vi "Config - access language vision ini file.vi"(5 ".ini Controller":enum16{"Read", "Write"}(ring), 6 "Language":T1, 8 "error in":errorcluster, 10 "English":T2={"Home"="Home", "Test Setup"="Setup", "Run Test"="Test", "Configure"="Config", "Hardware Viewer"="Viewer", "Review Test"="Review", "Report"="Folder Path:", "Exit"="Exit", "Device Connected?"="Device Connected?", "Test in Progress?"="Test in Progress?", "Simulate?"="Simulate?", "Device Type 1"="Corrugation Analysis Trolley", "Device Type 2"="Bi-Corrugation Analysis Trolley", "Device Type 3"="Bi-Corrugation Analysis Trolley", "Device Type 4"="Bi-Corrugation Analysis Trolley", "Device Type 5"="Bi-Corrugation Analysis Trolley", "Device Type 6"="Bi-Corrugation Analysis Trolley", "Device Type 7"="Bi-Corrugation Analysis Trolley", "Software Version"="Version", "Support"="Software by RailMeasurement Limited - Cambridge - UK - support@railmeasurement.com", "Operator"="Operator:", "Test Description"="Description:", "Line"="Description:", "Test Folder Path"="Folder Path:", "Test Folder Path RCA"="Folder Path:", "Start Position"="Start Position:", "Sensor Position"="Sensor Position:", "Sensor A Position"="Sensor A Position:", "Sensor B Position"="Sensor B Position:", "Visible Chart Distance"="Sensor B Position:", "Rail Side"="Rail Side:", "Rail A Side"="Rail A Side:", "Distance Direction"="Distance Direction:", "Start"="Start:", "Distance Travelled"="Distance Travelled:", "Current Position"="Current Position:", "Stop Test"="Stop", "Pause Test"="Save", "Displacement"="Displacement", "Position"="Position", "Sensor Calibration"="Sensor Calibration:", "Sensor A Calibration"="Sensor A Calibration:", "Sensor B Calibration"="Sensor B Calibration:", "Encoder Spacing"="Encoder Spacing:", "Sampling Distance"="Sampling Distance:", "Tacho Pulses/Rev"="Sensor Calibration:", "Wheel Diameter"="Sensor A Calibration:", "Sampling Distances"=["1mm", "2mm"], "Distance Unit"="Distance in:", "Distance Units"=["Kilometres", "miles & chains", "metres", "stations", "miles"], "Swap Direction"="Swap Direction at Run End?", "Language"="Language", "Device Resolution"="Save", "Device Resolutions"=["Kilometres", "miles & chains", "metres", "stations", "miles"], "Detect Change in Direction"="Save", "Save Config"="Save", "Encoder Data"="Encoder Data", "Sensor Data"="Sensor Data", "Sensor A Data"="Sensor A Data", "Sensor B Data"="Sensor B Data", "Voltage"="Voltage", "Time (m:s)"="Time (m:s)", "Unit mm/s/V"="(mm/s)/V", "Unit mm"="mm", "Unit km"="km", "Unit m"="m", "Start Test Message"="m", "Stop Test Message"="km", "Exit Message"="mm", "File Exists Message"="mm", "File Path Invalid Message"="mm", "Combine Error"="mm", "Combine Success"="mm", "Roller Comp Error"="mm", "Test Folder Path (Live)"="mm", "Folder Error"="Sensor B Position:", "Enc Count"="Setup", "Run Start"="mm", "Run End"="mm", "Date"="mm", "Train"="Sensor B Position:", "Location"="Setup", "Notes"="mm", "Heading_1"="mm", "Heading_2"="mm", "Left Rail"="Sensor B Position:", "Right Rail"="Setup", "Left Exclusions"="mm", "Right Exclusions"="mm", "Settings"="mm", "Wavelength Ranges"="Sensor B Position:", "Y-Axis Limits"="Setup", "Exc Limits"="Sensor B Position:", "Other Settings"="Setup", "Distance/Page"="mm", "Distance/Pages"=["Kilometres", "miles & chains", "metres", "stations", "miles"], "Gridlines"="mm", "Report Tolerance"="mm", "Manual Cut"="Sensor B Position:", "Plot Colour"="Distance in:", "Plot Colours"=["Kilometres", "miles & chains", "metres", "stations", "miles"], "EN Standard"="mm", "RiL Standard"="mm", "Custom Standard"="mm", "Resolution"="Distance in:", "Resolutions"=["Kilometres", "miles & chains", "metres", "stations", "miles"], "Exceedence Header"="mm", "Distance (km)"="mm", "Left (%)"="mm", "Right (%)"="Distance in:", "Page"="Distance in:", "Align"="mm", "Main"="mm", "Comparison"="Distance in:", "Offset"="Distance in:", "From"="Distance in:", "To"="Distance in:", "Of"="Distance in:", "File"="mm", "Load New"="mm", "Load Comparison"="Distance in:", "Discard Comparison"="Distance in:", "Print Current Page"="Distance in:", "Print All Pages"="Distance in:", "Print Exceedence Report"="Distance in:", "Plot Main"="Distance in:", "No Comparison Data to Align"="Distance in:", "Run Load Error"="Distance in:", "Report Load Error"="Distance in:", "Cut"="Distance in:", "Remove"="Distance in:", "Config Settings Unsaved"="Distance in:", "Acquisition Paused"="Distance in:", "Please Select One Option Below"="Distance in:", "RCA is Now Stationary"="Distance in:", "Reporting Setting"="Distance in:", "Main Abbreviated"="Distance in:", "Comparison Abbreviated"="Distance in:", "Exceedence Abbreviated"="Distance in:", "Align Comparison"="Distance in:", "Rail Corrugation Analyser Reporting"="Distance in:", "Show Exc. % in Graph"="Distance in:", "Evaluate Sections <100m"="Distance in:", "Evaluate Sections <0.062mile"="Distance in:", "Section Too Short for Evaluation"="Distance in:", "Language Change Prompt"="Distance in:", "Show All"="Distance in:", "Sections_km"="Distance in:", "Sections_mi"="Distance in:", "Vision"="Distance in:", "Vision Report"="Distance in:", "Vision Display"="Distance in:", "Vision Displays"=["Kilometres", "miles & chains", "metres", "stations", "miles"], "Save Images"="Distance in:", "Image Frequency"="Distance in:", "Section"="Distance in:", "Brightness"="Distance in:", "Contrast"="Distance in:", "Shadow"="Distance in:", "Sharpened"="Distance in:", "Apply to all Images"="Distance in:", "Reset"="Distance in:", "Are you sure"="Distance in:", "Image Processing"="Distance in:", "Save Video"="Distance in:", "Image Offset"="Distance in:", "Camera Mode"="Distance in:", "Camera Modes"=["Kilometres", "miles & chains", "metres", "stations", "miles"], "Copy Page"="Distance in:", "Copy Graphs"="Distance in:", "Camera Mode Change Prompt"="Distance in:", "Camera_1 Missing"="Distance in:", "Camera_2 Missing"="Distance in:", "Cameras Missing"="Distance in:", "Camera Setup"="Distance in:", "Camera_1 Connection Error"="Distance in:", "Camera_2 Connection Error"="Distance in:", "Cameras Connection Error"="Distance in:", "No GPS"="Distance in:", "No Signal"="Distance in:", "Camera_1 Connected"="Distance in:", "Camera_1 Not Connected"="Distance in:", "Camera_2 Connected"="Distance in:", "Camera_2 Not Connected"="Distance in:", "Start Position at 0m?"="Distance in:", "Continue"="Distance in:", "New Test, Same Direction"="Distance in:", "New Test, Opposite Direction"="Distance in:", "Stop and Save"="Distance in:", "Live Corrug Estimate"="Distance in:", "Wavelength Corrug"="Distance in:", "Distance Corrug "="Distance in:", "Update Corrug"="Distance in:", "Company"="Distance in:", "Ref Profile "="Distance in:", "Company_Report"="Distance in:", "Ref Profile_Report"="Distance in:", "Heading_1_RVHR"="Distance in:", "Heading_2_RVHR"="Distance in:", "Remove Feature"="Distance in:", "Feature Type"="Sampling Distance:", "Feature Types"=["1mm", "2mm"], "AI Not Ready"="Sampling Distance:"}, 11 "Config File Ref":T3=refnum) -> (0 "error out":errorcluster, 2 "HLC Controls Out":T2={"Home"="Home", "Test Setup"="Setup", "Run Test"="Test", "Configure"="Config", "Hardware Viewer"="Viewer", "Review Test"="Review", "Report"="Folder Path:", "Exit"="Exit", "Device Connected?"="Device Connected?", "Test in Progress?"="Test in Progress?", "Simulate?"="Simulate?", "Device Type 1"="Corrugation Analysis Trolley", "Device Type 2"="Bi-Corrugation Analysis Trolley", "Device Type 3"="Bi-Corrugation Analysis Trolley", "Device Type 4"="Bi-Corrugation Analysis Trolley", "Device Type 5"="Bi-Corrugation Analysis Trolley", "Device Type 6"="Bi-Corrugation Analysis Trolley", "Device Type 7"="Bi-Corrugation Analysis Trolley", "Software Version"="Version", "Support"="Software by RailMeasurement Limited - Cambridge - UK - support@railmeasurement.com", "Operator"="Operator:", "Test Description"="Description:", "Line"="Description:", "Test Folder Path"="Folder Path:", "Test Folder Path RCA"="Folder Path:", "Start Position"="Start Position:", "Sensor Position"="Sensor Position:", "Sensor A Position"="Sensor A Position:", "Sensor B Position"="Sensor B Position:", "Visible Chart Distance"="Sensor B Position:", "Rail Side"="Rail Side:", "Rail A Side"="Rail A Side:", "Distance Direction"="Distance Direction:", "Start"="Start:", "Distance Travelled"="Distance Travelled:", "Current Position"="Current Position:", "Stop Test"="Stop", "Pause Test"="Save", "Displacement"="Displacement", "Position"="Position", "Sensor Calibration"="Sensor Calibration:", "Sensor A Calibration"="Sensor A Calibration:", "Sensor B Calibration"="Sensor B Calibration:", "Encoder Spacing"="Encoder Spacing:", "Sampling Distance"="Sampling Distance:", "Tacho Pulses/Rev"="Sensor Calibration:", "Wheel Diameter"="Sensor A Calibration:", "Sampling Distances"=["1mm", "2mm"], "Distance Unit"="Distance in:", "Distance Units"=["Kilometres", "miles & chains", "metres", "stations", "miles"], "Swap Direction"="Swap Direction at Run End?", "Language"="Language", "Device Resolution"="Save", "Device Resolutions"=["Kilometres", "miles & chains", "metres", "stations", "miles"], "Detect Change in Direction"="Save", "Save Config"="Save", "Encoder Data"="Encoder Data", "Sensor Data"="Sensor Data", "Sensor A Data"="Sensor A Data", "Sensor B Data"="Sensor B Data", "Voltage"="Voltage", "Time (m:s)"="Time (m:s)", "Unit mm/s/V"="(mm/s)/V", "Unit mm"="mm", "Unit km"="km", "Unit m"="m", "Start Test Message"="m", "Stop Test Message"="km", "Exit Message"="mm", "File Exists Message"="mm", "File Path Invalid Message"="mm", "Combine Error"="mm", "Combine Success"="mm", "Roller Comp Error"="mm", "Test Folder Path (Live)"="mm", "Folder Error"="Sensor B Position:", "Enc Count"="Setup", "Run Start"="mm", "Run End"="mm", "Date"="mm", "Train"="Sensor B Position:", "Location"="Setup", "Notes"="mm", "Heading_1"="mm", "Heading_2"="mm", "Left Rail"="Sensor B Position:", "Right Rail"="Setup", "Left Exclusions"="mm", "Right Exclusions"="mm", "Settings"="mm", "Wavelength Ranges"="Sensor B Position:", "Y-Axis Limits"="Setup", "Exc Limits"="Sensor B Position:", "Other Settings"="Setup", "Distance/Page"="mm", "Distance/Pages"=["Kilometres", "miles & chains", "metres", "stations", "miles"], "Gridlines"="mm", "Report Tolerance"="mm", "Manual Cut"="Sensor B Position:", "Plot Colour"="Distance in:", "Plot Colours"=["Kilometres", "miles & chains", "metres", "stations", "miles"], "EN Standard"="mm", "RiL Standard"="mm", "Custom Standard"="mm", "Resolution"="Distance in:", "Resolutions"=["Kilometres", "miles & chains", "metres", "stations", "miles"], "Exceedence Header"="mm", "Distance (km)"="mm", "Left (%)"="mm", "Right (%)"="Distance in:", "Page"="Distance in:", "Align"="mm", "Main"="mm", "Comparison"="Distance in:", "Offset"="Distance in:", "From"="Distance in:", "To"="Distance in:", "Of"="Distance in:", "File"="mm", "Load New"="mm", "Load Comparison"="Distance in:", "Discard Comparison"="Distance in:", "Print Current Page"="Distance in:", "Print All Pages"="Distance in:", "Print Exceedence Report"="Distance in:", "Plot Main"="Distance in:", "No Comparison Data to Align"="Distance in:", "Run Load Error"="Distance in:", "Report Load Error"="Distance in:", "Cut"="Distance in:", "Remove"="Distance in:", "Config Settings Unsaved"="Distance in:", "Acquisition Paused"="Distance in:", "Please Select One Option Below"="Distance in:", "RCA is Now Stationary"="Distance in:", "Reporting Setting"="Distance in:", "Main Abbreviated"="Distance in:", "Comparison Abbreviated"="Distance in:", "Exceedence Abbreviated"="Distance in:", "Align Comparison"="Distance in:", "Rail Corrugation Analyser Reporting"="Distance in:", "Show Exc. % in Graph"="Distance in:", "Evaluate Sections <100m"="Distance in:", "Evaluate Sections <0.062mile"="Distance in:", "Section Too Short for Evaluation"="Distance in:", "Language Change Prompt"="Distance in:", "Show All"="Distance in:", "Sections_km"="Distance in:", "Sections_mi"="Distance in:", "Vision"="Distance in:", "Vision Report"="Distance in:", "Vision Display"="Distance in:", "Vision Displays"=["Kilometres", "miles & chains", "metres", "stations", "miles"], "Save Images"="Distance in:", "Image Frequency"="Distance in:", "Section"="Distance in:", "Brightness"="Distance in:", "Contrast"="Distance in:", "Shadow"="Distance in:", "Sharpened"="Distance in:", "Apply to all Images"="Distance in:", "Reset"="Distance in:", "Are you sure"="Distance in:", "Image Processing"="Distance in:", "Save Video"="Distance in:", "Image Offset"="Distance in:", "Camera Mode"="Distance in:", "Camera Modes"=["Kilometres", "miles & chains", "metres", "stations", "miles"], "Copy Page"="Distance in:", "Copy Graphs"="Distance in:", "Camera Mode Change Prompt"="Distance in:", "Camera_1 Missing"="Distance in:", "Camera_2 Missing"="Distance in:", "Cameras Missing"="Distance in:", "Camera Setup"="Distance in:", "Camera_1 Connection Error"="Distance in:", "Camera_2 Connection Error"="Distance in:", "Cameras Connection Error"="Distance in:", "No GPS"="Distance in:", "No Signal"="Distance in:", "Camera_1 Connected"="Distance in:", "Camera_1 Not Connected"="Distance in:", "Camera_2 Connected"="Distance in:", "Camera_2 Not Connected"="Distance in:", "Start Position at 0m?"="Distance in:", "Continue"="Distance in:", "New Test, Same Direction"="Distance in:", "New Test, Opposite Direction"="Distance in:", "Stop and Save"="Distance in:", "Live Corrug Estimate"="Distance in:", "Wavelength Corrug"="Distance in:", "Distance Corrug "="Distance in:", "Update Corrug"="Distance in:", "Company"="Distance in:", "Ref Profile "="Distance in:", "Company_Report"="Distance in:", "Ref Profile_Report"="Distance in:", "Heading_1_RVHR"="Distance in:", "Heading_2_RVHR"="Distance in:", "Remove Feature"="Distance in:", "Feature Type"="Sampling Distance:", "Feature Types"=["1mm", "2mm"], "AI Not Ready"="Sampling Distance:"}, 3 "refnum out":T3)   [LabVIEW 2023]
doc: "This subVI reads initial config data from a .ini file to define the default UI.\n\nAuthor: D Keeling\nDate: 20/05/2012\nVersion: 1.0"
uses:
  <vilib>/Utility/config.llb/NI_LVConfig.lvlib
  <vilib>/Utility/config.llb/Config Data RefNum.ctl
  Controls/Language.ctl
  Controls/Language Vision Text Cluster.ctl
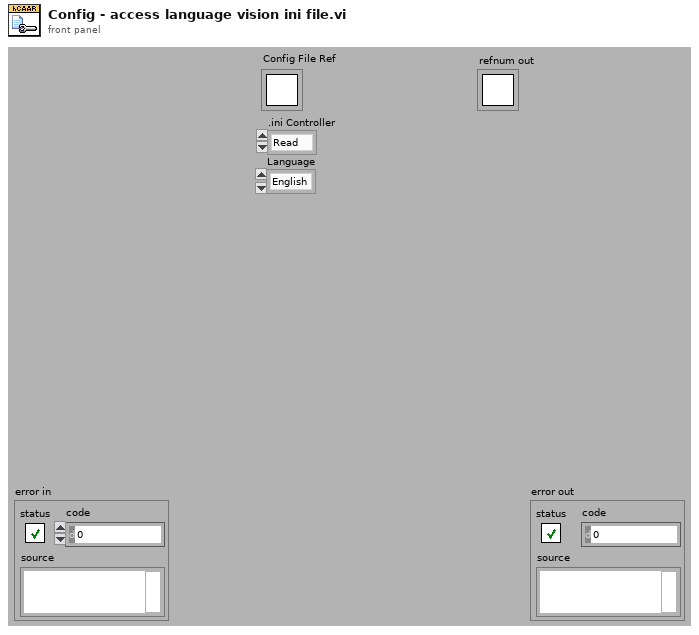
[diagram p1: front panel]
types:
  T1 = typedef "Language.ctl" = enum16{"English", "Chinese", "German"}
  T2 = typedef "Language Vision Text Cluster.ctl" = cluster{"Home":string, "Test Setup":string, "Run Test":string, "Configure":string, "Hardware Viewer":string, "Review Test":string, "Report":string, "Exit":string, "Device Connected?":string, "Test in Progress?":string, "Simulate?":string, "Device Type 1":string, "Device Type 2":string, "Device Type 3":string, "Device Type 4":string, "Device Type 5":string, "Device Type 6":string, "Device Type 7":string, "Software Version":string, "Support":string, "Operator":string, "Test Description":string, "Line":string, "Test Folder Path":string, "Test Folder Path RCA":string, "Start Position":string, "Sensor Position":string, "Sensor A Position":string, "Sensor B Position":string, "Visible Chart Distance":string, "Rail Side":string, "Rail A Side":string, "Distance Direction":string, "Start":string, "Distance Travelled":string, "Current Position":string, "Stop Test":string, "Pause Test":string, "Displacement":string, "Position":string, "Sensor Calibration":string, "Sensor A Calibration":string, "Sensor B Calibration":string, "Encoder Spacing":string, "Sampling Distance":string, "Tacho Pulses/Rev":string, "Wheel Diameter":string, "Sampling Distances":string[], "Distance Unit":string, "Distance Units":string[], "Swap Direction":string, "Language":string, "Device Resolution":string, "Device Resolutions":string[], "Detect Change in Direction":string, "Save Config":string, "Encoder Data":string, "Sensor Data":string, "Sensor A Data":string, "Sensor B Data":string, "Voltage":string, "Time (m:s)":string, "Unit mm/s/V":string, "Unit mm":string, "Unit km":string, "Unit m":string, "Start Test Message":string, "Stop Test Message":string, "Exit Message":string, "File Exists Message":string, "File Path Invalid Message":string, "Combine Error":string, "Combine Success":string, "Roller Comp Error":string, "Test Folder Path (Live)":string, "Folder Error":string, "Enc Count":string, "Run Start":string, "Run End":string, "Date":string, "Train":string, "Location":string, "Notes":string, "Heading_1":string, "Heading_2":string, "Left Rail":string, "Right Rail":string, "Left Exclusions":string, "Right Exclusions":string, "Settings":string, "Wavelength Ranges":string, "Y-Axis Limits":string, "Exc Limits":string, "Other Settings":string, "Distance/Page":string, "Distance/Pages":string[], "Gridlines":string, "Report Tolerance":string, "Manual Cut":string, "Plot Colour":string, "Plot Colours":string[], "EN Standard":string, "RiL Standard":string, "Custom Standard":string, "Resolution":string, "Resolutions":string[], "Exceedence Header":string, "Distance (km)":string, "Left (%)":string, "Right (%)":string, "Page":string, "Align":string, "Main":string, "Comparison":string, "Offset":string, "From":string, "To":string, "Of":string, "File":string, "Load New":string, "Load Comparison":string, "Discard Comparison":string, "Print Current Page":string, "Print All Pages":string, "Print Exceedence Report":string, "Plot Main":string, "No Comparison Data to Align":string, "Run Load Error":string, "Report Load Error":string, "Cut":string, "Remove":string, "Config Settings Unsaved":string, "Acquisition Paused":string, "Please Select One Option Below":string, "RCA is Now Stationary":string, "Reporting Setting":string, "Main Abbreviated":string, "Comparison Abbreviated":string, "Exceedence Abbreviated":string, "Align Comparison":string, "Rail Corrugation Analyser Reporting":string, "Show Exc. % in Graph":string, "Evaluate Sections <100m":string, "Evaluate Sections <0.062mile":string, "Section Too Short for Evaluation":string, "Language Change Prompt":string, "Show All":string, "Sections_km":string, "Sections_mi":string, "Vision":string, "Vision Report":string, "Vision Display":string, "Vision Displays":string[], "Save Images":string, "Image Frequency":string, "Section":string, "Brightness":string, "Contrast":string, "Shadow":string, "Sharpened":string, "Apply to all Images":string, "Reset":string, "Are you sure":string, "Image Processing":string, "Save Video":string, "Image Offset":string, "Camera Mode":string, "Camera Modes":string[], "Copy Page":string, "Copy Graphs":string, "Camera Mode Change Prompt":string, "Camera_1 Missing":string, "Camera_2 Missing":string, "Cameras Missing":string, "Camera Setup":string, "Camera_1 Connection Error":string, "Camera_2 Connection Error":string, "Cameras Connection Error":string, "No GPS":string, "No Signal":string, "Camera_1 Connected":string, "Camera_1 Not Connected":string, "Camera_2 Connected":string, "Camera_2 Not Connected":string, "Start Position at 0m?":string, "Continue":string, "New Test, Same Direction":string, "New Test, Opposite Direction":string, "Stop and Save":string, "Live Corrug Estimate":string, "Wavelength Corrug":string, "Distance Corrug ":string, "Update Corrug":string, "Company":string, "Ref Profile ":string, "Company_Report":string, "Ref Profile_Report":string, "Heading_1_RVHR":string, "Heading_2_RVHR":string, "Remove Feature":string, "Feature Type":string, "Feature Types":string[], "AI Not Ready":string}
  T3 = typedef "NI_LVConfig.lvlib/Config Data RefNum.ctl" = refnum<k1>
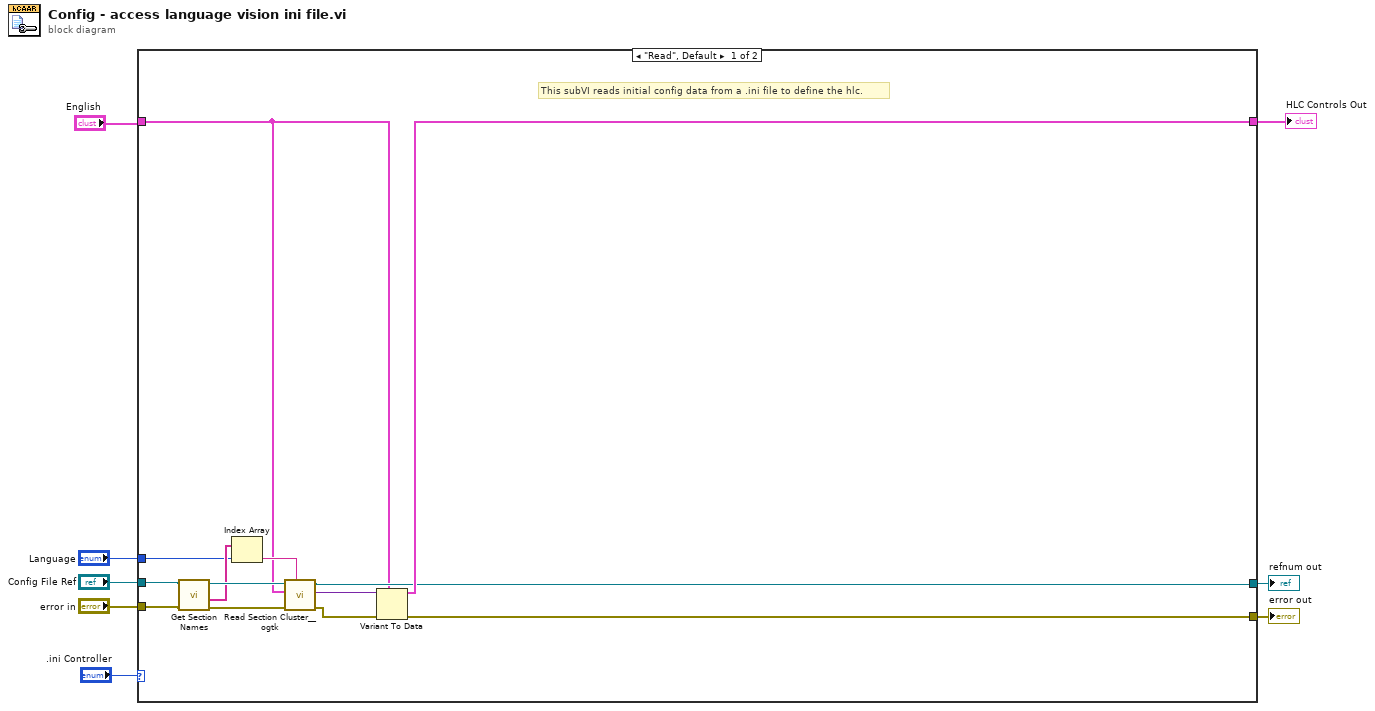
[diagram p0: block diagram]
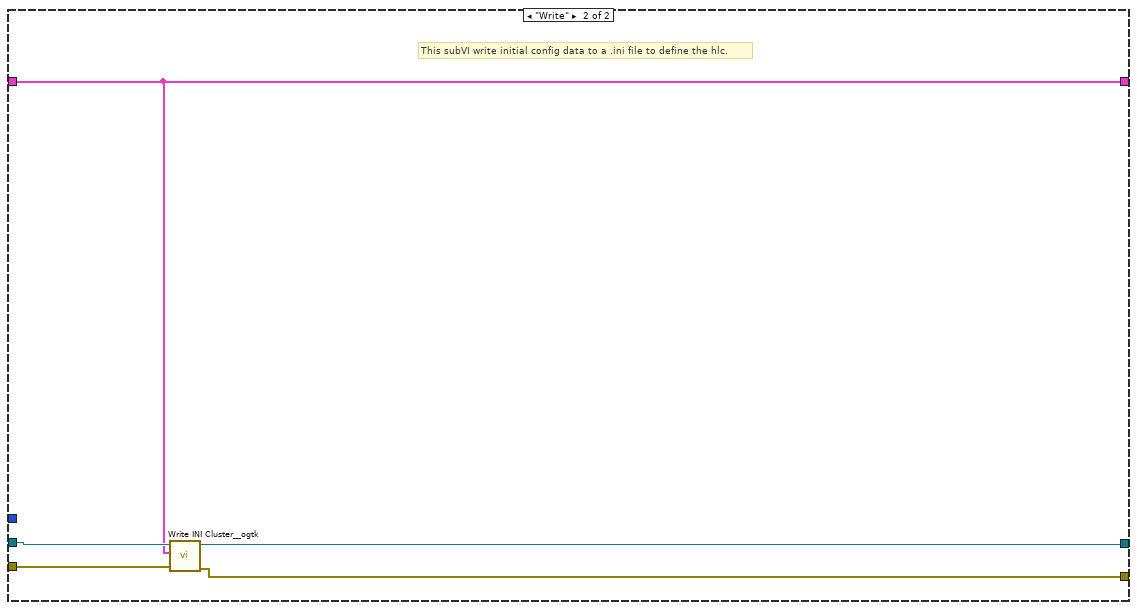
[diagram p2: hidden frame]
diagram:
  n1 = case shown="\"Read\", Default" ".ini Controller" {
    tunnel: [w21 w26] -> w7
    tunnel: "Config File Ref" -> [w14 w23]
    tunnel: [w11 w25] -> w6
    tunnel: "English" -> [w10 w22]
    tunnel: [w20 w22] -> w5
    tunnel: "error in" -> [w15 w24]
    tunnel: "Language" -> [w9 _]
    frame "Read", Default {
      # "This subVI reads initial config data from a .ini file to define the hlc."
      n2 = call <vilib>:"Get Section Names.vi"("error in (no error)"=w15, "refnum"=w14) -> ("error out"=w19:errorcluster, "section names"=w17:string[], "refnum out"=w18:T3)  [unwired: 7 in]
      n3 = Index Array(array=w17, index=w9) -> (element=w16:string)
      n4 = call "Read Section Cluster__ogtk.vi"("section (optional)"=w16, "error in (no error)"=w19, "Section Formatted Cluster Type"=w10, "refnum"=w18) -> ("error out"=w13:errorcluster, "Section Formatted Cluster"=w12:variant, "dup refnum"=w11:T3)  [unwired: 3 in, 2 out]
      n5 = Variant To Data(error in=w13, type=w10, Variant=w12) -> (data=w20:T2, error out=w21:errorcluster)
    }
    frame "Write" {
      # "This subVI write initial config data to a .ini file to define the hlc."
      n6 = call "Write INI Cluster__ogtk.vi"("error in (no error)"=w24, "INI Fomatted Cluster"=w22, "refnum"=w23) -> ("error out"=w26:errorcluster, "dup refnum"=w25:T3)  [unwired: 7 in]
    }
  }
  "error out" <- w7
  "refnum out" <- w6
  "HLC Controls Out" <- w5
